vi "Create Tree.vi"(8 "error in (no error)":errorcluster, 10 "Tree Refnum":refnum<vi>, 11 "Tree Name":string) -> (0 "error out":errorcluster, 3 "Tree_LVOOP out":refnum<class "Tree Class.lvclass">)   [LabVIEW 2012, in "Tree Tools.lvlib" / "Tree Class.lvclass"]
uses:
  Tree Class.lvclass
  Tree Tag Class/Tree Tag Class.lvclass
  Tree Class.lvclass/Tree Class.ctl
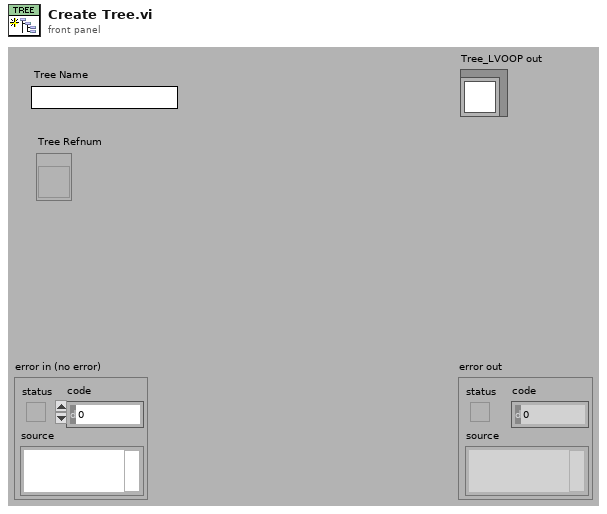
[diagram p1: front panel]
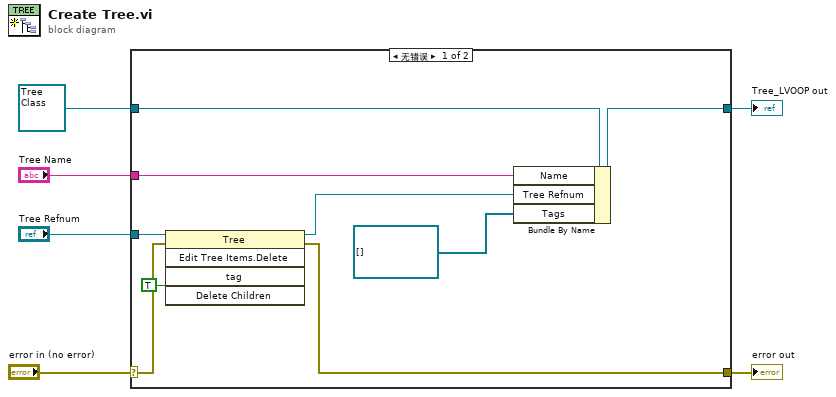
[diagram p0: block diagram]
diagram:
  n1 = case shown="无错误" "error in (no error)" {
    selector: "error in (no error)" -> [w9 w17]
    tunnel: [w8 w17] -> w5
    tunnel: [w14 w16] -> w3
    tunnel: refnum<class "Tree Class.lvclass"> refnum ("Tree_LVOOP in") -> [w15 w16]
    tunnel: "Tree Name" -> [w13 _]
    tunnel: "Tree Refnum" -> [w12 _]
    frame No Error {
      n2 = invoke class="Tree" method="Edit Tree Items.Delete"(reference=w12, error in=w9, "Delete Children"=TRUE ("Delete Children?")) -> (reference out=w10:refnum<vi>, error out=w8:errorcluster)  [unwired: 2 in, 3 out]
      n3 = Bundle By Name(cluster=w15, "Name"=w13, "Tree Refnum"=w10, "Tags"=refnum<class "Tree Tag Class.lvclass">[] []) -> (w14:refnum<class "Tree Class.lvclass">)
    }
    frame Error {
    }
  }
  "error out" <- w5
  "Tree_LVOOP out" <- w3
